vi "Get File Extension from Name String.vi"(0 "File Name String":string) -> (1 "filename without extension":string, 2 "lowercase file extension":string)   [LabVIEW 2014]
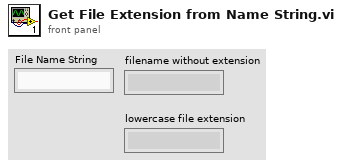
[diagram p1: front panel]
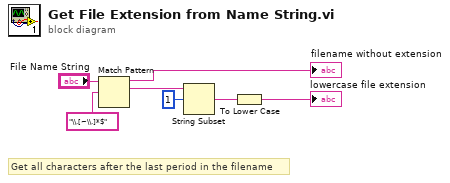
[diagram p0: block diagram]
diagram:
  # "Get all characters after the last period in the filename"
  n1 = Match Pattern(string="File Name String", regular expression="\\.[~\\.]*$") -> (before substring=→"filename without extension":string, match substring=w5:string)  [unwired: 3 out]
  n2 = String Subset(string=w5, offset (0)=1) -> (substring=w4:string)  [unwired: 1 out]
  n3 = To Lower Case(string=w4) -> (all lower case string=→"lowercase file extension":string)
